vi "习题7.1.vi"() -> ()   [LabVIEW 2017]
uses:
  <vilib>/measure/NI_MABase.lvlib
panel:
  out "XY图":cluster{"Y":dbl[], "Y":dbl[]}(graph)
  in  "phase 2":dbl caption="相位" format="%.2p"
  in  "amplitude 2":dbl=1.0 caption="幅值" format="%0.2p"
  in  "frequency 2":dbl=10.0 caption="频率" format="%0.2p"
  in  "phase":dbl caption="相位" format="%.2p"
  in  "amplitude":dbl=1.0 caption="幅值" format="%0.2p"
  in  "frequency":dbl=10.0 caption="频率" format="%0.2p"
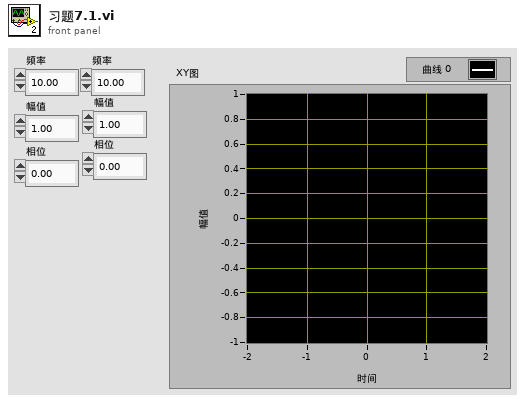
[diagram p1: front panel]
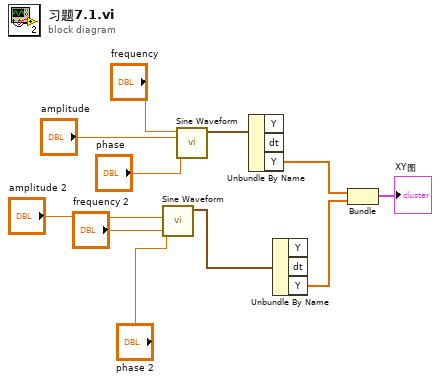
[diagram p0: block diagram]
diagram:
  n1 = call <vilib>:"Sine Waveform.vi"("phase"="phase 2", "amplitude"="amplitude 2", "frequency"="frequency 2") -> ("signal out"=w10:waveform(dbl))  [unwired: 7 in, 1 out]
  n2 = call <vilib>:"Sine Waveform.vi"("phase"="phase", "amplitude"="amplitude", "frequency"="frequency") -> ("signal out"=w11:waveform(dbl))  [unwired: 7 in, 1 out]
  n3 = Unbundle By Name(w11) -> ("Y"=w4:dbl[])  [unwired: 2 out]
  n4 = Unbundle By Name(w10) -> ("Y"=w3:dbl[])  [unwired: 2 out]
  n5 = Bundle("Y"=w4, "Y"=w3) -> (→"XY图":cluster{"Y":dbl[], "Y":dbl[]})  [unwired: 1 in]
